vi "CameraReader.vi"(2 "file path (dialog if empty)":path=path "C:/Program Files (x86)/FRC Dashboard", 3 "name or relative path":string="Blue.csv") -> (0 "User Settings":T1, 1 "Camera Settings":T2)   [LabVIEW 2013]
uses:
  <vilib>/Utility/file.llb/Read From Spreadsheet File (string).vi
panel:
  out "SteadyTime":dbl
  out "TargetMarMin":dbl
  out "TargetMarMax":dbl
  out "Color":u16
  out "AngM":dbl
  out "CamB":dbl
  out "CamM":dbl
  out "Dadj":dbl
  out "Radj":dbl
  out "Ladj":dbl
  out "CamW":dbl
  out "RFOV":dbl
  out "LFOV":dbl
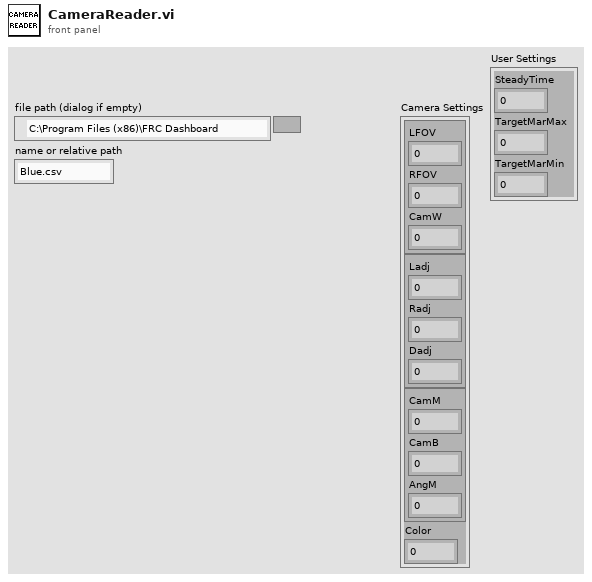
[diagram p1: front panel]
types:
  T1 = cluster{"SteadyTime":dbl, "TargetMarMax":dbl, "TargetMarMin":dbl}
  T2 = cluster{cluster{"LFOV":dbl, "RFOV":dbl, "CamW":dbl}, cluster{"Ladj":dbl, "Radj":dbl, "Dadj":dbl}, cluster{"CamM":dbl, "CamB":dbl, "AngM":dbl}, "Color":u16}
  T3 = cluster{"all rows[0]":string, "all rows[1]":string, "all rows[2]":string, "all rows[3]":string, "all rows[4]":string, "all rows[5]":string, "all rows[6]":string, "all rows[7]":string, "all rows[8]":string}
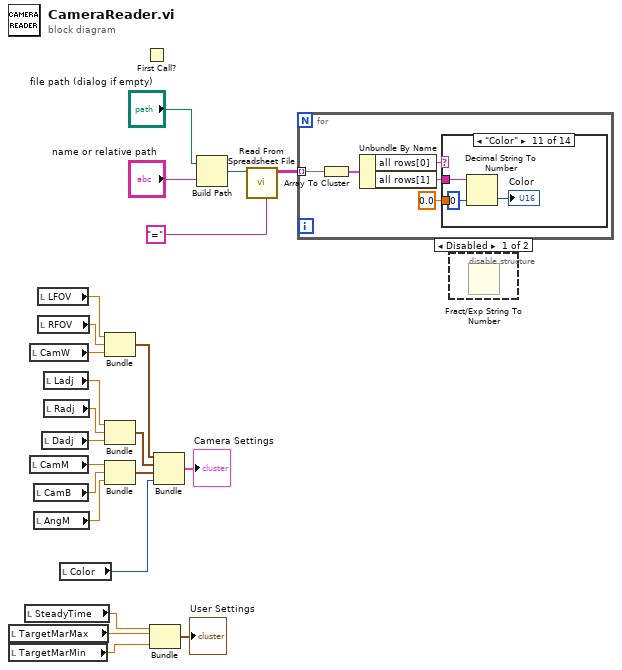
[diagram p0: block diagram]
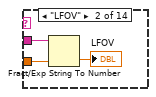
[diagram p4: hidden frame]
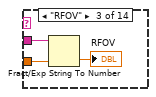
[diagram p5: hidden frame]
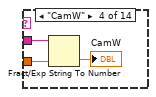
[diagram p6: hidden frame]
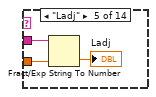
[diagram p7: hidden frame]
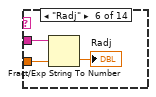
[diagram p8: hidden frame]
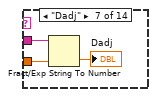
[diagram p9: hidden frame]
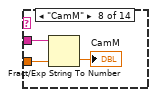
[diagram p10: hidden frame]
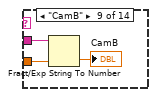
[diagram p11: hidden frame]
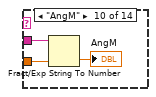
[diagram p12: hidden frame]
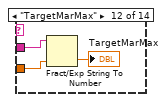
[diagram p13: hidden frame]
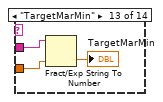
[diagram p14: hidden frame]
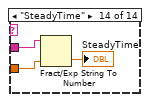
[diagram p15: hidden frame]
diagram:
  n1 = local read "TargetMarMax"() -> (w3:dbl)
  n2 = local read "TargetMarMin"() -> (w2:dbl)
  n3 = local read "SteadyTime"() -> (w4:dbl)
  n4 = local read "CamW"() -> (w14:dbl)
  n5 = local read "CamM"() -> (w12:dbl)
  n6 = local read "CamB"() -> (w11:dbl)
  n7 = local read "AngM"() -> (w10:dbl)
  n8 = local read "LFOV"() -> (w17:dbl)
  n9 = local read "RFOV"() -> (w13:dbl)
  n10 = local read "Dadj"() -> (w15:dbl)
  n11 = local read "Ladj"() -> (w18:dbl)
  n12 = local read "Radj"() -> (w16:dbl)
  n13 = local read "Color"() -> (w6:u16)
  n14 = Bundle("LFOV"=w17, "RFOV"=w13, "CamW"=w14) -> (w19:cluster{"LFOV":dbl, "RFOV":dbl, "CamW":dbl})  [unwired: 1 in]
  n15 = Bundle("Ladj"=w18, "Radj"=w16, "Dadj"=w15) -> (w20:cluster{"Ladj":dbl, "Radj":dbl, "Dadj":dbl})  [unwired: 1 in]
  n16 = Bundle("CamM"=w12, "CamB"=w11, "AngM"=w10) -> (w9:cluster{"CamM":dbl, "CamB":dbl, "AngM":dbl})  [unwired: 1 in]
  n17 = First Call?() -> ()  [unwired: 1 out]
  n18 = Bundle("SteadyTime"=w4, "TargetMarMax"=w3, "TargetMarMin"=w2) -> (→"User Settings":T1)  [unwired: 1 in]
  n19 = Bundle(w19, w20, w9, "Color"=w6) -> (→"Camera Settings":T2)  [unwired: 1 in]
  n20 = Build Path(base path="file path (dialog if empty)", name or relative path="name or relative path") -> (appended path=w7:path)
  n21 = call-poly <vilib>:"Read From Spreadsheet File.vi"("delimiter (\\t)"="=", "file path (dialog if empty)"=w7) -> ("all rows"=w8:string[][])  [unwired: 5 in, 4 out]
  n22 = for {
    tunnel: w8 -> [w28] mode=indexing
    n23 = Array To Cluster(array=w28) -> (cluster=w27:T3)
    n24 = Unbundle By Name(w27) -> ("all rows[0]"=w26:string, "all rows[1]"=w25:string)
    n25 = case shown="\"Color\"" w26 {
      tunnel: w25 -> [_ w31 w34 w37 w40 w43 w46 w49 w52 w55 w58 w60 w63 w66]
      tunnel: 0.0 ("default (0 I32)") -> [_ w29 w32 w35 w38 w41 w44 w47 w50 w53 _ w59 w62 w65]
      frame "", Default {
      }
      frame "LFOV" {
        n26 = Fract/Exp String To Number(string=w31, default (0 dbl)=w29) -> (number=→"LFOV":dbl)  [unwired: 2 in, 1 out]
      }
      frame "RFOV" {
        n27 = Fract/Exp String To Number(string=w34, default (0 dbl)=w32) -> (number=→"RFOV":dbl)  [unwired: 2 in, 1 out]
      }
      frame "CamW" {
        n28 = Fract/Exp String To Number(string=w37, default (0 dbl)=w35) -> (number=→"CamW":dbl)  [unwired: 2 in, 1 out]
      }
      frame "Ladj" {
        n29 = Fract/Exp String To Number(string=w40, default (0 dbl)=w38) -> (number=→"Ladj":dbl)  [unwired: 2 in, 1 out]
      }
      frame "Radj" {
        n30 = Fract/Exp String To Number(string=w43, default (0 dbl)=w41) -> (number=→"Radj":dbl)  [unwired: 2 in, 1 out]
      }
      frame "Dadj" {
        n31 = Fract/Exp String To Number(string=w46, default (0 dbl)=w44) -> (number=→"Dadj":dbl)  [unwired: 2 in, 1 out]
      }
      frame "CamM" {
        n32 = Fract/Exp String To Number(string=w49, default (0 dbl)=w47) -> (number=→"CamM":dbl)  [unwired: 2 in, 1 out]
      }
      frame "CamB" {
        n33 = Fract/Exp String To Number(string=w52, default (0 dbl)=w50) -> (number=→"CamB":dbl)  [unwired: 2 in, 1 out]
      }
      frame "AngM" {
        n34 = Fract/Exp String To Number(string=w55, default (0 dbl)=w53) -> (number=→"AngM":dbl)  [unwired: 2 in, 1 out]
      }
      frame "Color" {
        n35 = Decimal String To Number(string=w58, default (0L)=u16 0 ("default (0 I32)")) -> (number=→"Color":u16)  [unwired: 1 in, 1 out]
      }
      frame "TargetMarMax" {
        n36 = Fract/Exp String To Number(string=w60, default (0 dbl)=w59) -> (number=→"TargetMarMax":dbl)  [unwired: 2 in, 1 out]
      }
      frame "TargetMarMin" {
        n37 = Fract/Exp String To Number(string=w63, default (0 dbl)=w62) -> (number=→"TargetMarMin":dbl)  [unwired: 2 in, 1 out]
      }
      frame "SteadyTime" {
        n38 = Fract/Exp String To Number(string=w66, default (0 dbl)=w65) -> (number=→"SteadyTime":dbl)  [unwired: 2 in, 1 out]
      }
    }
  }
  n39 = disable-structure shown="Disabled" {
    frame Disabled {
      n40 = Fract/Exp String To Number() -> ()  [unwired: 4 in, 2 out]
    }
    frame Enabled {
    }
  }
